vi "Git_GetHeadBody.vi"(4 "Your Password (not necessary)":string, 6 "Your User Name (not necessary)":string, 8 "error in (no error)":errorcluster, 10 "timeout (10000)":i32=10000, 11 "Address":string) -> (0 "error out":errorcluster, 2 "body":string, 3 "headers":string)   [LabVIEW 2012]
doc: "This is a low level VI which contacts the GitHub api, to get the info for a given address. The username and password are imbedded into the https address."
uses:
  <vilib>/httpClient/LabVIEWHTTPClient.lvlib
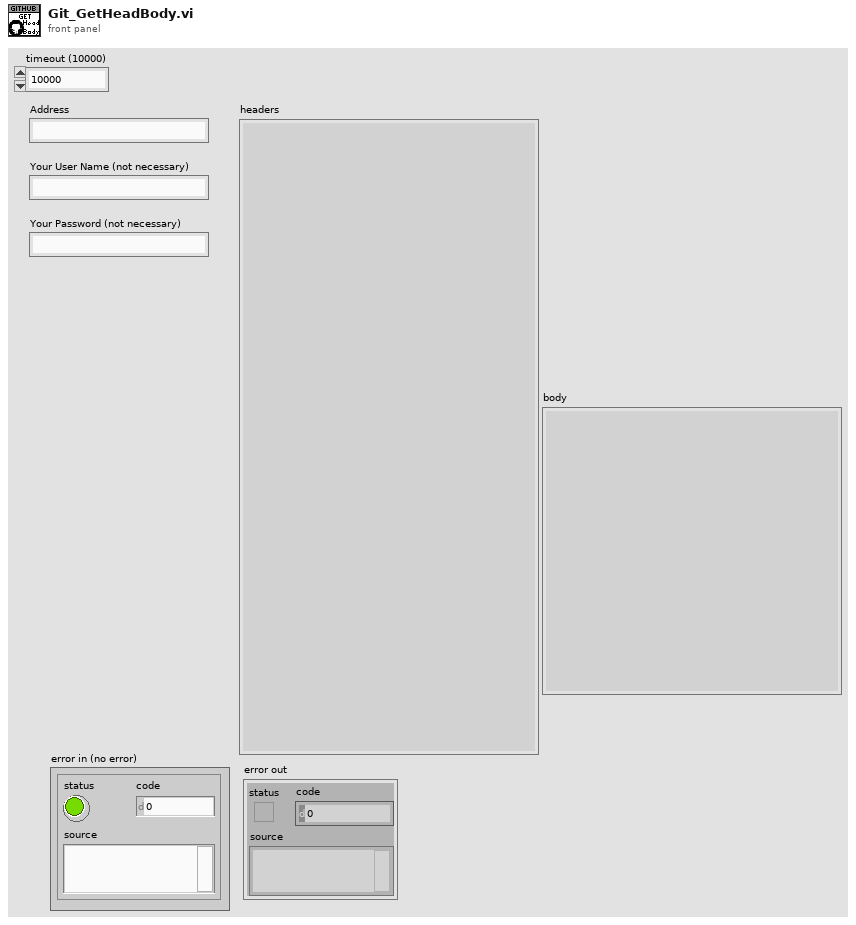
[diagram p1: front panel]
types:
  T1 = typedef "LabVIEWHTTPClient.lvlib/ClientHandle.ctl" = refnum<k1>
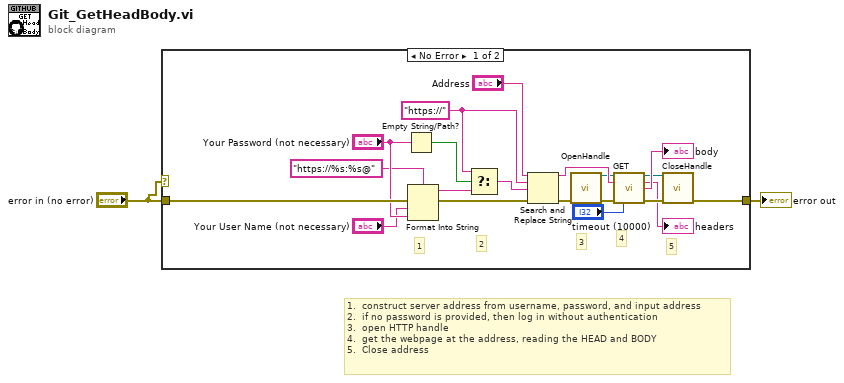
[diagram p0: block diagram]
diagram:
  # "1.  construct server address from username, password, and input address\n2.  if no password is provided, then log in without authentication\n3.  open HTTP handle\n4.  get the webpage at the address, reading the HEAD and BODY\n5.  Close address"
  n1 = case shown="No Error" "error in (no error)" {
    tunnel: "error in (no error)" -> [w22 w23]
    tunnel: [w21 w23] -> w2
    frame No Error {
      w13 = "https://" ("search string")
      # "5"
      # "4"
      # "3"
      # "2"
      # "1"
      n2 = Empty String/Path?(string/path="Your Password (not necessary)") -> (empty?=w12:bool)
      n3 = Format Into String(format string="https://%s:%s@", error in=w22, "Your User Name (not necessary)", "Your Password (not necessary)") -> (resulting string=w14:string, error out=w19:errorcluster)  [unwired: 1 in]
      n4 = Select(t=w13, s=w12, f=w14) -> (s? t:f=w15:string)
      n5 = Search and Replace String(input string="Address", search string=w13, replace string=w15, error in=w19) -> (result string=w20:string, error out=w18:errorcluster)  [unwired: 4 in, 2 out]
      n6 = call <vilib>:"OpenHandle.vi"("error in (no error)"=w18) -> ("client handle out"=w17:T1, "error out"=w16:errorcluster)  [unwired: 13 in]
      n7 = call <vilib>:"GET.vi"("client handle"=w17, "url"=w20, "error in (no error)"=w16, "timeout (10000)"="timeout (10000)") -> ("client handle out"=w4:T1, "headers"=→"headers":string, "body"=→"body":string, "error out"=w6:errorcluster)  [unwired: 8 in]
      n8 = call <vilib>:"CloseHandle.vi"("client handle"=w4, "error in (no error)"=w6) -> ("error out"=w21:errorcluster)  [unwired: 13 in]
    }
    frame Error {
    }
  }
  "error out" <- w2
